vi "Username Prompt.vi"(10 "Password":string, 11 "Username":string) -> (2 "Password out":string, 3 "Username out":string)   [LabVIEW 2014, in "Spark API.lvlib"]
uses:
  Spark API.lvlib
panel:
  in  "Log In":bool
  # "Please enter a valid username and password for Spark.io"
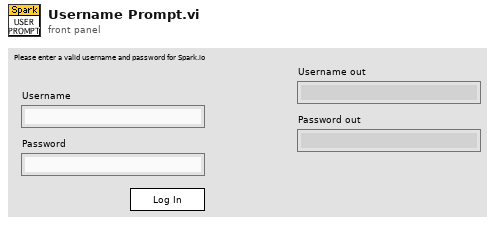
[diagram p1: front panel]
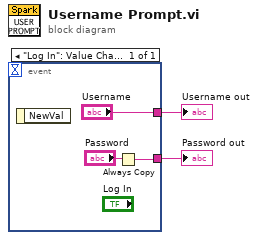
[diagram p0: block diagram]
diagram:
  n1 = event shown="[0] \"Log In\": Value Change" {
    selector: _ -> [_]
    dyn-events: _ -> [_]
    timeout: _ -> [_]
    tunnel: ["Username"] -> w2
    tunnel: [w3] -> w1
    event "Log In": Value Change {
      n2 = event-data() -> ()  [unwired: 1 in, 1 out]
      n3 = Always Copy(1:"Password") -> (0:w3:string)
    }
  }
  "Password out" <- w1
  "Username out" <- w2
